vi "Build Tree.vi"(8 "error in (no error)":errorcluster, 9 "No Project Text Reference":refnum<vi>, 10 "Tree Reference In":refnum<vi>, 11 "CS++MessageMakerMain in":refnum<class "CS++MessageMakerMain.lvclass">) -> (0 "error out":errorcluster, 2 "Tree Reference Out":refnum<vi>, 3 "CS++MessageMakerMain out":refnum<class "CS++MessageMakerMain.lvclass">)   [LabVIEW 2014, in "CS++MessageMakerMain.lvlib" / "CS++MessageMakerMain.lvclass"]
doc: "Updates the Tree on the Front Panel."
uses:
  CS++MessageMakerMain.lvclass
  CS++MessageMakerMain.lvclass/CS++MessageMakerMain.ctl
  CSPP_Actor/CS++Actor.lvclass/CS++Actor.ctl
  CSPP_Method/CS++Method.lvclass/CS++Method.ctl
  CSPP_Message/CS++Message.lvclass/CS++Message.ctl
  CSPP_Actor/CS++Actor.lvclass
  CSPP_Method/CS++Method.lvclass
  CSPP_Message/CS++Message.lvclass
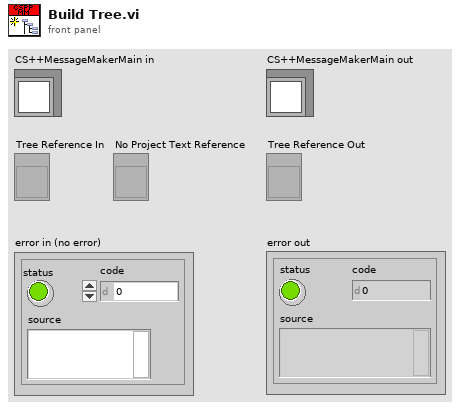
[diagram p1: front panel]
types:
  T1 = cluster{"Left Cell String":string, "Child Text":string[], "Child Tag":string, "Item Indent":i32, "Child Only?":bool, "Glyph Index":i32}
  T2 = typedef "CS++Message.lvlib/CS++Message.lvclass/MessageStatus.ctl" = u16
  T3 = cluster{"Left Cell String":string, "Child Text":string[], "Child Tag":string, "Item Indent":i32, "Child Only?":bool, "Glyph Index":i32}[]
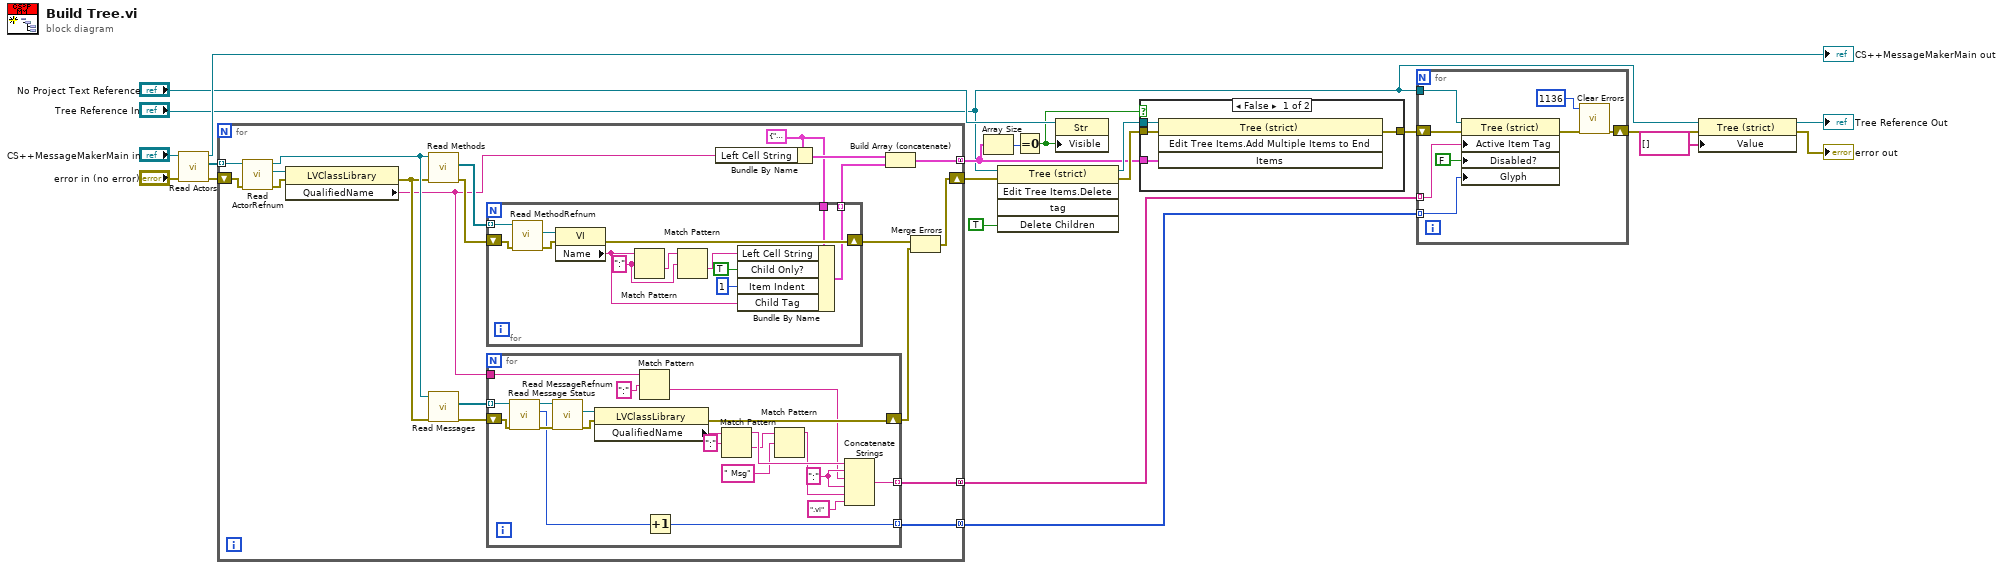
[diagram p0: block diagram]
diagram:
  n1 = call "Read Actors.vi"("error in (no error)"="error in (no error)", "CS++MessageMakerMain in"="CS++MessageMakerMain in") -> ("error out"=w20:errorcluster, "Actors"=w21:refnum<class "CS++Actor.lvclass">[], "CS++MessageMakerMain out"=→"CS++MessageMakerMain out":refnum<class "CS++MessageMakerMain.lvclass">)  [unwired: 7 in]
  n2 = for {
    tunnel: w21 -> [w39] mode=indexing
    shift-right: [w23] -> w18
    shift-left: w20 -> [w40]
    tunnel: [w33] -> w16 mode=concatenating
    tunnel: [w26] -> w12 mode=concatenating
    tunnel: [w22] -> w1 mode=concatenating
    w34 = T1 {"Left Cell String"="", "Child Text"=[], "Child Tag"="", "Item Indent"=0, "Child Only?"=FALSE, "Glyph Index"=0} ("Item")
    n3 = call "Read ActorRefnum.vi"("error in (no error)"=w40, "CS++Actor in"=w39) -> ("error out"=w37:errorcluster, "ActorRefnum"=w38:refnum<vi>, "CS++Actor out"=w31:refnum<class "CS++Actor.lvclass">)  [unwired: 7 in]
    n4 = property class="LVClassLibrary"(reference=w38, error in=w37) -> (error out=w30:errorcluster, "QualifiedName"=w27:string)  [unwired: 1 out]
    n5 = call "Read Methods.vi"("error in (no error)"=w30, "CS++Actor in"=w31) -> ("error out"=w36:errorcluster, "Methods"=w35:refnum<class "CS++Method.lvclass">[])  [unwired: 7 in, 1 out]
    n6 = call "Read Messages.vi"("error in (no error)"=w30, "CS++Actor in"=w31) -> ("error out"=w28:errorcluster, "Messages"=w29:refnum<class "CS++Message.lvclass">[])  [unwired: 7 in, 1 out]
    n7 = for {
      shift-right: [w71] -> w25
      shift-left: w36 -> [w75]
      tunnel: w35 -> [w74] mode=indexing
      tunnel: w34 -> [w70]
      tunnel: [w67] -> w32 mode=indexing
      w65 = ":"
      n8 = call "Read MethodRefnum.vi"("error in (no error)"=w75, "CS++Methods in"=w74) -> ("error out"=w72:errorcluster, "MethodRefnum"=w73:refnum<vi>)  [unwired: 7 in, 1 out]
      n9 = property class="VI"(reference=w73, error in=w72) -> (error out=w71:errorcluster, "Name"=w63:string)  [unwired: 1 out]
      n10 = Match Pattern(string=w63, regular expression=w65) -> (after substring=w66:string)  [unwired: 1 in, 3 out]
      n11 = Match Pattern(string=w66, regular expression=w65) -> (after substring=w64:string)  [unwired: 1 in, 3 out]
      n12 = Bundle By Name(cluster=w70, "Left Cell String"=w64, "Child Only?"=TRUE, "Item Indent"=1, "Child Tag"=w63) -> (w67:T1)
    }
    n13 = for {
      tunnel: w29 -> [w47] mode=indexing
      shift-right: [w60] -> w24
      shift-left: w28 -> [w45]
      tunnel: w27 -> [w54]
      tunnel: [w56] -> w26 mode=indexing
      tunnel: [w42] -> w22 mode=indexing
      w49 = ":" ("string")
      n14 = call "Read Message Status.vi"("error in (no error)"=w45, "CS++Message in"=w47) -> ("error out"=w44:errorcluster, "Message Status"=w43:T2, "CS++Message out"=w46:refnum<class "CS++Message.lvclass">)  [unwired: 7 in]
      n15 = call "Read MessageRefnum.vi"("error in (no error)"=w44, "CS++Message in"=w46) -> ("error out"=w61:errorcluster, "MessageRefnum"=w62:refnum<vi>)  [unwired: 7 in, 1 out]
      n16 = property class="LVClassLibrary"(reference=w62, error in=w61) -> (error out=w60:errorcluster, "QualifiedName"=w58:string)  [unwired: 1 out]
      n17 = Match Pattern(string=w54, regular expression=":") -> (after substring=w48:string)  [unwired: 1 in, 3 out]
      n18 = Increment(x=w43) -> (x+1=w42:T2)
      n19 = Match Pattern(string=w58, regular expression=":") -> (before substring=w57:string, after substring=w51:string)  [unwired: 1 in, 2 out]
      n20 = Match Pattern(string=w51, regular expression=" Msg") -> (before substring=w50:string)  [unwired: 1 in, 3 out]
      n21 = Concatenate Strings(w57, w49, w48, w49, w50, ".vi" ("string")) -> (w56:string)
    }
    n22 = Bundle By Name(cluster=w34, "Left Cell String"=w27) -> (w41:T1)
    n23 = Build Array (concatenate)(w41, w32) -> (w33:T3)
    n24 = Merge Errors(w25, w24) -> (w23:errorcluster)
  }
  n25 = Array Size(array=w16) -> (size(s)=w15:i32)
  n26 = invoke class="Tree (strict)" method="Edit Tree Items.Delete"(reference="Tree Reference In", error in=w18, "Delete Children"=TRUE ("Delete Children?")) -> (reference out=w19:refnum<vi>, error out=w17:errorcluster)  [unwired: 2 in, 3 out]
  n27 = Equal To 0?(x=w15) -> (x = 0?=w4:bool)
  n28 = property on="Property Node" class="Str"(reference="No Project Text Reference", "Visible"=w4) -> ()  [unwired: 1 in, 2 out]
  n29 = case shown="False" w4 {
    tunnel: w19 -> [w79 _]
    tunnel: w17 -> [w78 w80]
    tunnel: w16 -> [w77 _]
    tunnel: [w76 w80] -> w13
    frame False {
      n30 = invoke on="Invoke Node" class="Tree (strict)" method="Edit Tree Items.Add Multiple Items to End"(reference=w79, error in=w78, "Items"=w77) -> (error out=w76:errorcluster)  [unwired: 1 in, 3 out]
    }
    frame True {
    }
  }
  n31 = for {
    shift-right: [w83] -> w7
    shift-left: w13 -> [w86]
    tunnel: w12 -> [w87] mode=indexing
    tunnel: "Tree Reference In" -> [w85]
    tunnel: w1 -> [w81] mode=indexing
    n32 = property class="Tree (strict)"(reference=w85, error in=w86, "Active Item Tag"=w87, "Disabled?"=FALSE ("Active Item:Disabled?"), "Glyph"=w81) -> (error out=w84:errorcluster)  [unwired: 1 out]
    n33 = call <vilib>:"Clear Errors.vi"("error in (no error)"=w84, "specific error code to clear (0: all)"=1136) -> ("error out"=w83:errorcluster)  [unwired: 4 in, 1 out]
  }
  n34 = property class="Tree (strict)"(reference="Tree Reference In", error in=w7, "Value"=string[] []) -> (reference out=→"Tree Reference Out":refnum<vi>, error out=→"error out":errorcluster)
